vi "Launch New Network Connection.vi"(5 "Handler VI ref":T1, 6 "FPGA Ref":T2, 7 "Listener ID":refnum<k5>, 8 "error in (no error)":errorcluster, 9 "Remote Port":u16, 10 "Remote Address":string, 11 "Connection ID":refnum<k5>) -> (0 "error out":errorcluster, 2 "conn ID Out":refnum<k5>, 3 "Handler VI Ref out":T1)   [LabVIEW 2020]
doc: "Author: Scott Hannahs <sth@magnet.fsu.edu>\nCopyright 2018 Florida State University, All rights reserved."
uses:
  RT Controls/FPGA SCH Digitizer Ref.ctl
  Net Conn Handler VI.ctl
  RT Controls/Network Info.ctl
  RT Controls/RT System Auth Level.ctl
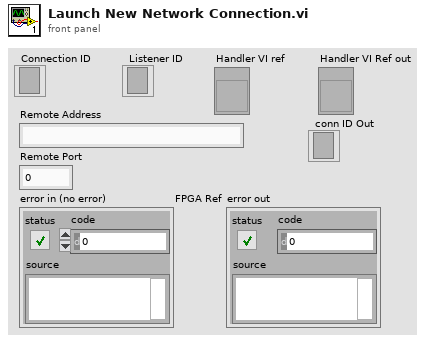
[diagram p1: front panel]
types:
  T1 = typedef "Net Conn Handler VI.ctl" = refnum<vi>
  T2 = typedef "FPGA SCH Digitizer Ref.ctl" = refnum<k20>
  T3 = typedef "Network Info.ctl" = cluster{"Listener ID":refnum<k5>, "Connection ID":refnum<k5>, "Remote Address":string, "Remote Port":u16, "DataLoc":u32, "RawData":cluster{"#Pts":u32, "Pointer":u32}, "Last Comm Time":timestamp, "Authorized":T4}
  T4 = typedef "RT System Auth Level.ctl" = enum16{"Read Only", "Operator", "Admin"}
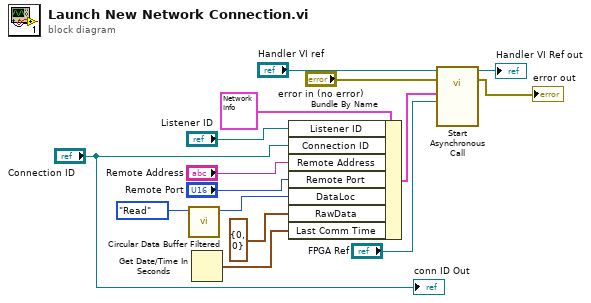
[diagram p0: block diagram]
diagram:
  n1 = call "Circular Data Buffer Filtered.vi"("Action"=enum16{"Initialize", "Write", "Read", "Clear"}."Read" ("Enum")) -> ("Next Write"=w6:u32)  [unwired: 8 in, 2 out]
  n2 = Get Date/Time In Seconds() -> (seconds since 1Jan1904=w15:timestamp)
  n3 = Bundle By Name(cluster=T3 {"Listener ID"=refnum, "Connection ID"=refnum, "Remote Address"="", "Remote Port"=0, "DataLoc"=0, "RawData"={"#Pts"=0, "Pointer"=0}, "Last Comm Time"=timestamp(0 s since 1904-01-01), "Authorized"=enum."Read Only"}, "Listener ID"="Listener ID", "Connection ID"="Connection ID", "Remote Address"="Remote Address", "Remote Port"="Remote Port", "DataLoc"=w6, "RawData"=cluster{"#Pts":u32, "Pointer":u32} {"#Pts"=0, "Pointer"=0}, "Last Comm Time"=w15) -> (w9:T3)
  n4 = call-by-ref "Start Asynchronous Call"(reference="Handler VI ref", error in="error in (no error)", "FPGA Ref"="FPGA Ref", "Network Info"=w9) -> (reference out=→"Handler VI Ref out":T1, error out=→"error out":errorcluster)  [unwired: 8 in, 2 out]
  "conn ID Out" <- "Connection ID"
